vi "write_params.vi"(8 "error in (no error)":errorcluster, 10 "params":T1={"n_components"={"n_components_type"="None", "n_components_int"=0.0}, "alpha"=1.0, "ridge_alpha"=0.01, "max_iter"=1000.0, "tol"=1e-08, "method"="lars", "n_jobs"=1.0, "U_init"={"U_init_type"="None", "U_init_list"=[]}, "V_init"={"V_init_type"="None", "V_init_list"=[]}, "verbose"=0.0, "random_state"=0.0}, 11 "SparsePCA in":refnum<class "SparsePCA.lvclass">) -> (0 "error out":errorcluster, 3 "SparsePCA out":refnum<class "SparsePCA.lvclass">)   [LabVIEW 2020, in "SparsePCA.lvclass"]
uses:
  SparsePCA.lvclass
  Controls/sparse_pca_params.ctl
  SparsePCA.lvclass/SparsePCA.ctl
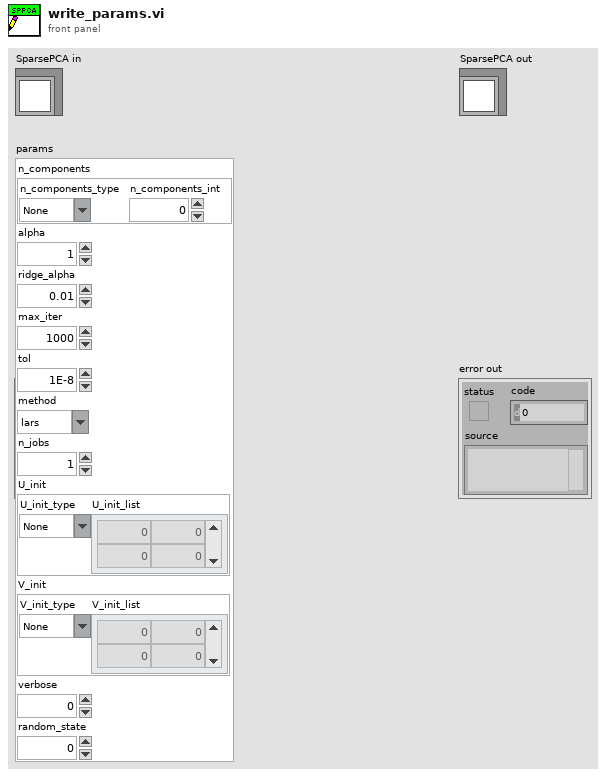
[diagram p1: front panel]
types:
  T1 = typedef "sparse_pca_params.ctl" = cluster{"n_components":cluster{"n_components_type":string, "n_components_int":dbl}, "alpha":dbl, "ridge_alpha":dbl, "max_iter":dbl, "tol":dbl, "method":string, "n_jobs":dbl, "U_init":cluster{"U_init_type":string, "U_init_list":dbl[][]}, "V_init":cluster{"V_init_type":string, "V_init_list":dbl[][]}, "verbose":dbl, "random_state":dbl}
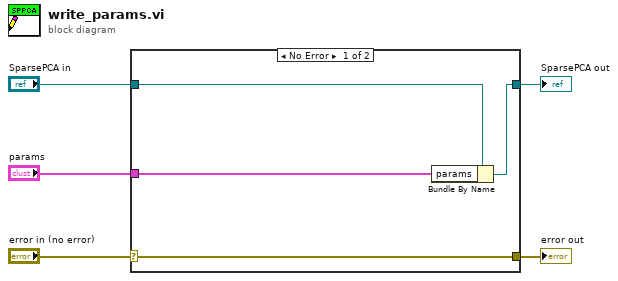
[diagram p0: block diagram]
diagram:
  n1 = case shown="No Error" "error in (no error)" {
    selector: "error in (no error)" -> [w9 w10]
    tunnel: [w9 w10] -> w4
    tunnel: [w7 w11] -> w2
    tunnel: "SparsePCA in" -> [w8 w11]
    tunnel: "params" -> [w6 _]
    frame No Error {
      n2 = Bundle By Name(cluster=w8, "params"=w6) -> (w7:refnum<class "SparsePCA.lvclass">)
    }
    frame Error {
    }
  }
  "error out" <- w4
  "SparsePCA out" <- w2
